vi "pull test data(com).vi"(8 "error in":errorcluster, 11 "VISA resource name in":refnum<visa-resource-name>) -> (0 "error out":errorcluster, 2 "received array":u8[](array[numeric]), 3 "VISA resource name out":refnum<visa-resource-name>)   [LabVIEW 2017, in "SPELS test.lvlib"]
uses:
  SPELS test.lvlib
panel:
  out "return count":u32
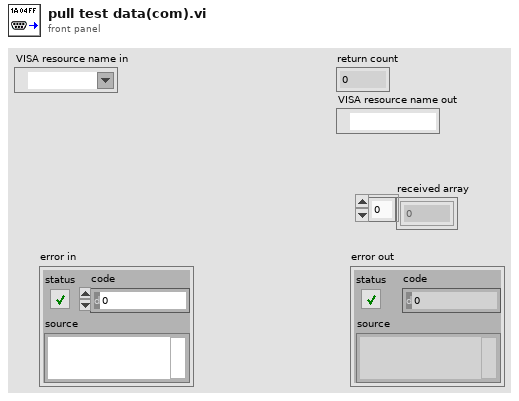
[diagram p1: front panel]
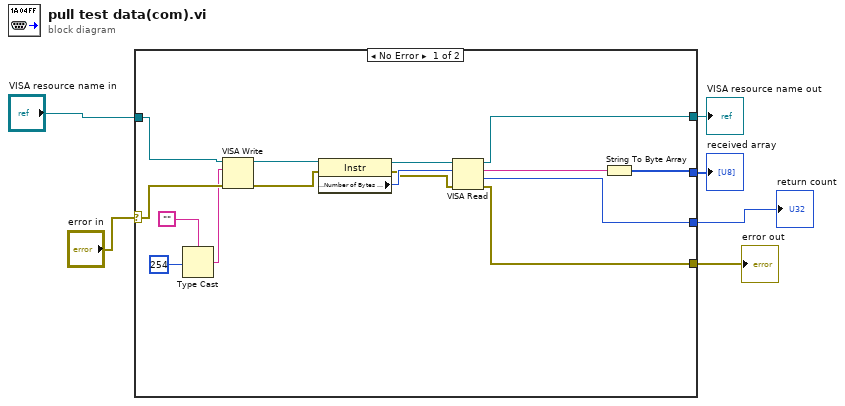
[diagram p0: block diagram]
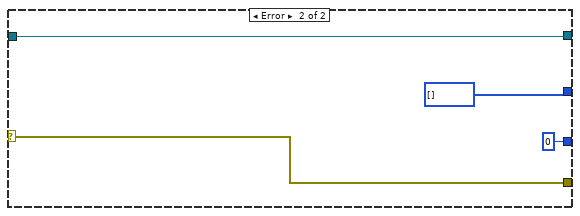
[diagram p2: hidden frame]
diagram:
  n1 = case shown="No Error" "error in" {
    selector: "error in" -> [w13 w25]
    tunnel: [w19 w25] -> w5
    tunnel: [w21 u8[] [] ("unsigned byte array")] -> w4
    tunnel: [w18 u32 0 ("return count")] -> w3
    tunnel: [w17 w22] -> w1
    tunnel: "VISA resource name in" -> [w10 w22]
    frame No Error {
      n2 = Type Cast(type="", x=u8 254) -> (*(type *) &x=w7:string)
      n3 = VISA Write(VISA resource name=w10, write buffer=w7, error in (no error)=w13) -> (VISA resource name out=w11:refnum<visa-resource-name>, error out=w12:errorcluster)  [unwired: 1 out]
      n4 = property class="Instr"(reference=w11, error in=w12) -> (reference out=w14:refnum<visa-resource-name>, error out=w15:errorcluster, "Serial Settings:Number of Bytes at Serial Port"=w16:u32)
      n5 = VISA Read(VISA resource name=w14, byte count=w16, error in (no error)=w15) -> (VISA resource name out=w17:refnum<visa-resource-name>, read buffer=w20:string, return count=w18:u32, error out=w19:errorcluster)
      n6 = String To Byte Array(string=w20) -> (unsigned byte array=w21:u8[])
    }
    frame Error {
    }
  }
  "error out" <- w5
  "received array" <- w4
  "return count" <- w3
  "VISA resource name out" <- w1
